vi "Path_Support Directory.vi"() -> (3 "Support Directory":path)   [LabVIEW 2023]
uses:
  <userlib>/_OpenG.lib/file/file.llb/openg_file.lvlib
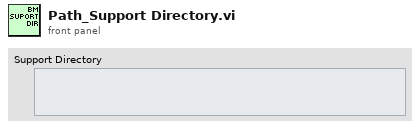
[diagram p1: front panel]
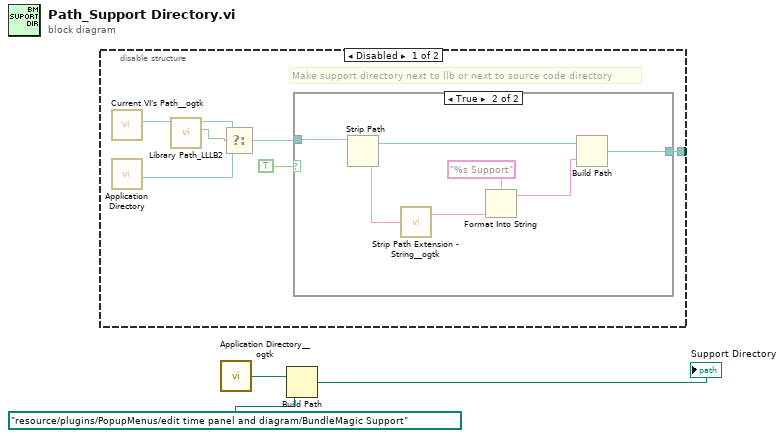
[diagram p0: block diagram]
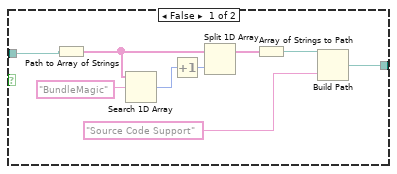
[diagram p2: hidden frame]
diagram:
  n1 = disable-structure shown="Disabled" {
    disable-tunnel: [w10 _] -> _
    frame Disabled {
      # "Make support directory next to llb or next to source code directory"
      n2 = call <userlib>:"Current VI's Path__ogtk.vi"() -> ("Current VI's Path (+ Relative)"=w7:path)  [unwired: 1 in]
      n3 = call <vilib>:"Application Directory.vi"() -> ("Application Directory"=w9:path)
      n4 = call "Library Path_LLLB2.vi"("File Path"=w7) -> ("Is in llb?"=w5:bool, "llb path"=w6:path)  [unwired: 9 in]
      n5 = Select(t=w6, s=w5, f=w9) -> (s? t:f=w8:path)
      n6 = case shown="True" TRUE {
        tunnel: [w12 w21] -> w10
        tunnel: w8 -> [w19 w20]
        frame False {
          n7 = Path to Array of Strings(0:w19) -> (2:w17:string[])  [unwired: 1 out]
          n8 = Search 1D Array(1D array=w17, element="BundleMagic") -> (index of element=w16:i32)  [unwired: 1 in]
          n9 = Increment(x=w16) -> (x+1=w11:i32)
          n10 = Split 1D Array(array=w17, index=w11) -> (first subarray=w15:string[])  [unwired: 1 out]
          n11 = Array of Strings to Path(0:w15) -> (2:w14:path)  [unwired: 1 in]
          n12 = Build Path(base path=w14, name or relative path="Source Code Support" ("element")) -> (appended path=w12:path)
        }
        frame True {
          n13 = Strip Path(path=w20) -> (stripped path=w26:path, name=w25:string)
          n14 = call <userlib>:"Strip Path Extension - String__ogtk.vi"("path"=w25) -> ("root"=w24:string)  [unwired: 1 out]
          n15 = Format Into String(format string="%s Support", w24) -> (resulting string=w22:string)  [unwired: 2 in, 1 out]
          n16 = Build Path(base path=w26, name or relative path=w22) -> (appended path=w21:path)
        }
      }
    }
    frame Enabled {
    }
  }
  n17 = call <userlib>:"Application Directory__ogtk.vi"() -> ("Application Directory (+ Relative)"=w1:path)  [unwired: 1 in]
  n18 = Build Path(base path=w1, name or relative path=path "resource/plugins/PopupMenus/edit time panel and diagram/BundleMagic Support" ("Support Directory")) -> (appended path=→"Support Directory":path)
